vi "Play Item Score.vi"(4 "Play Item":T1) -> (1 "Score":u32)   [LabVIEW 2020, in "AoC 2022.lvlib"]
uses:
  AoC 2022.lvlib
  Play Item.ctl
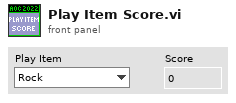
[diagram p1: front panel]
types:
  T1 = typedef "AoC 2022.lvlib/Play Item.ctl" = enum16{"Rock", "Paper", "Scissor"}
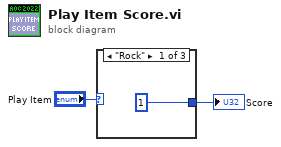
[diagram p0: block diagram]
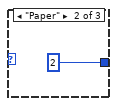
[diagram p2: hidden frame]
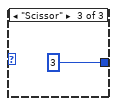
[diagram p3: hidden frame]
diagram:
  n1 = case shown="\"Rock\"" "Play Item" {
    tunnel: [u32 1 u32 2 u32 3] -> w2
    frame "Rock" {
    }
    frame "Paper" {
    }
    frame "Scissor" {
    }
  }
  "Score" <- w2
